vi "channeldata_complexsingle_interleaved.vi"() -> ()   [LabVIEW 2019]
panel:
  out "Error Out":errorcluster
  in  "TDMS File":path=path "C:/Python/projects/nitdms/tests/tdms_files/channeldata_complexsingle_interleaved.tdms"
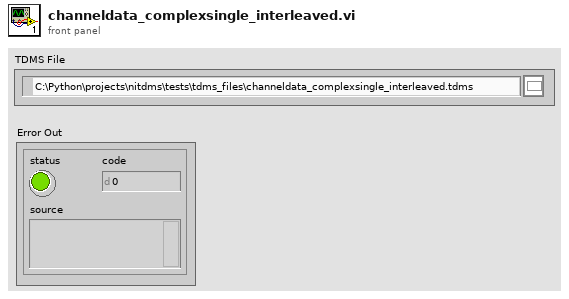
[diagram p1: front panel]
types:
  T1 = enum16{"open", "open or create", "create or replace", "create", "open (read-only)"}
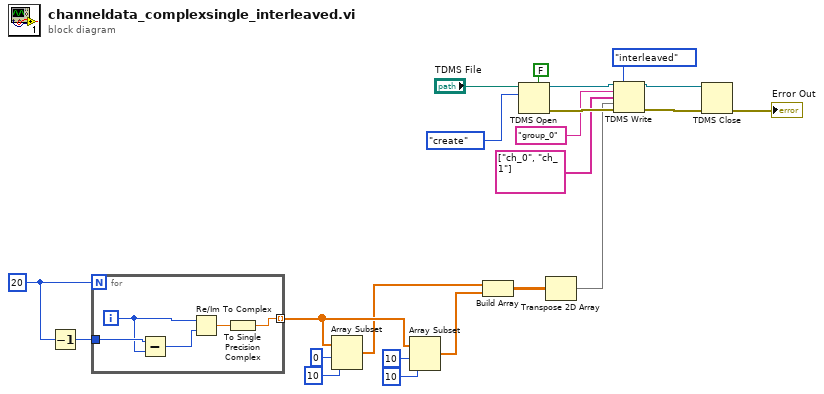
[diagram p0: block diagram]
diagram:
  w3 = 20
  n1 = Decrement(x=w3) -> (x-1=w2:i32)
  n2 = for {
    N: w3 -> [_]
    tunnel: [w23] -> w6 mode=indexing
    tunnel: w2 -> [w27]
    i -> [w26]
    n3 = Subtract(x=w27, y=w26) -> (x-y=w25:i32)
    n4 = Re/Im To Complex(1:w25, 2:w26) -> (0:w24:cdb)
    n5 = To Single Precision Complex(1:w24) -> (0:w23:csg)
  }
  n6 = Array Subset(array=w6, index=0, length=10) -> (w5:csg[])
  n7 = Array Subset(array=w6, index=10, length=10) -> (w4:csg[])
  n8 = Build Array(w5, w4) -> (w1:csg[][])
  n9 = TDMS Open(5:FALSE ("create index file? (T)"), 10:T1."create" ("operation (0:open)"), 11:"TDMS File") -> (0:w18:errorcluster, 3:w17:refnum<k34>)  [unwired: 4 in]
  n10 = Transpose 2D Array(2D array=w1) -> (transposed array=w11:csg[][])
  n11 = TDMS Write(0:w17, 1:enum16{"decimated", "interleaved"}."interleaved" ("data layout (0:decimated)"), 5:"group_0", 7:string[] ["ch_0", "ch_1"], 9:w11, 11:w18) -> (4:w15:refnum<k34>, 15:w16:errorcluster)  [unwired: 2 out]
  n12 = TDMS Close(8:w16, 11:w15) -> (0:→"Error Out":errorcluster)  [unwired: 1 out]
